vi "Command (read & write) - DI.vi"(7 "timeout ms (100)":i32=100, 8 "error in (no error)":errorcluster, 9 "Distance / Position":i32=-2147483648, 10 "IP":string, 11 "connection ID in":refnum<k16>) -> (0 "error out":errorcluster, 2 "Distance / Position":i32, 3 "connection ID out":refnum<k16>)   [LabVIEW 2016, in "SMD-7615.lvlib" / "eSCL.lvlib"]
doc: "DI - Distance/Position\nSets or requests the move distance in encoder counts (servo) or steps (stepper). The sign of DI indicates move direction: no sign means CW and “-” means CCW. DI sets both the distance for relative moves, like FL, and the position for absolute moves, like FP. DI also sets the direction of rotation for jogging (CJ)."
uses:
  eSCL.lvlib
  I32 Command and Param.ctl
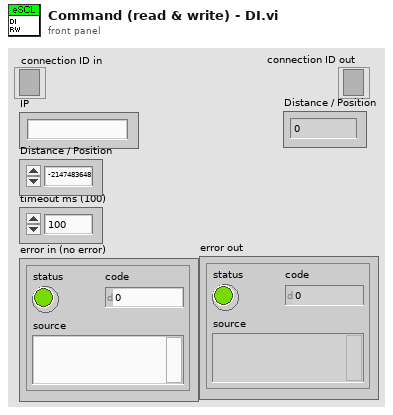
[diagram p1: front panel]
types:
  T1 = typedef "SMD-7615.lvlib/eSCL.lvlib/I32 Command and Param.ctl" = cluster{"Command":string, "I32 Parameler":i32, "I32 Parameler Default":i32, "I32 Parameler Coerece Upper":i32, "I32 Parameler Coerece Lower":i32}
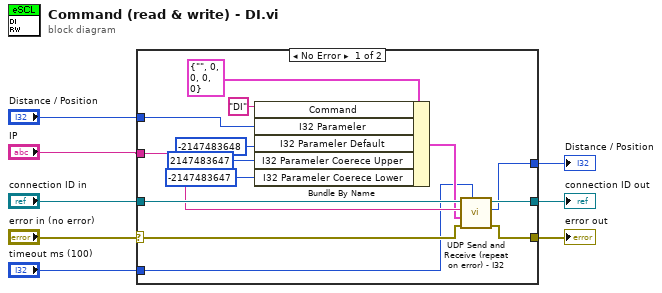
[diagram p0: block diagram]
diagram:
  n1 = case shown="No Error" "error in (no error)" {
    selector: "error in (no error)" -> [w14 w23]
    tunnel: "connection ID in" -> [w17 w24]
    tunnel: [w12 w24] -> w2
    tunnel: [w11 w23] -> w1
    tunnel: "IP" -> [w16 _]
    tunnel: "timeout ms (100)" -> [w13 _]
    tunnel: [w10 _] -> w3
    tunnel: "Distance / Position" -> [w18 _]
    frame No Error {
      n2 = Bundle By Name(cluster=T1 {"Command"="", "I32 Parameler"=0, "I32 Parameler Default"=0, "I32 Parameler Coerece Upper"=0, "I32 Parameler Coerece Lower"=0} ("I32 Command & Param"), "Command"="DI", "I32 Parameler"=w18, "I32 Parameler Default"=-2147483648 ("DBL Parameler Default"), "I32 Parameler Coerece Upper"=2147483647 ("DBL Parameler Coerece Upper"), "I32 Parameler Coerece Lower"=-2147483647 ("DBL Parameler Coerece Lower")) -> (w15:T1)
      n3 = call "UDP Send and Receive (repeat on error) - I32.vi"("timeout ms (100)"=w13, "error in (no error)"=w14, "I32 Command & Param"=w15, "IP"=w16, "connection ID in"=w17) -> ("error out"=w11:errorcluster, "DBL Param out"=w10:i32, "connection ID out"=w12:refnum<k16>)  [unwired: 4 in]
    }
    frame Error {
    }
  }
  "connection ID out" <- w2
  "error out" <- w1
  "Distance / Position" <- w3
